vi "Service Stop Handler.vi"(8 "error in":errorcluster, 9 "stop server user event":T1, 10 "stop button ref":refnum<vi>, 11 "measurement service in":refnum<class "IMeasurement Service.lvclass">) -> (0 "error out":errorcluster, 3 "measurement service out":refnum<class "IMeasurement Service.lvclass">)   [LabVIEW 2020, in "NI Measurement Plug-In SDK.lvlib" / "IMeasurement Service.lvclass"]
uses:
  IMeasurement Service.lvclass
  Helpers/TypeDefs/Stop Server User Event.ctl
  NI Measurement Plug-In SDK.lvlib
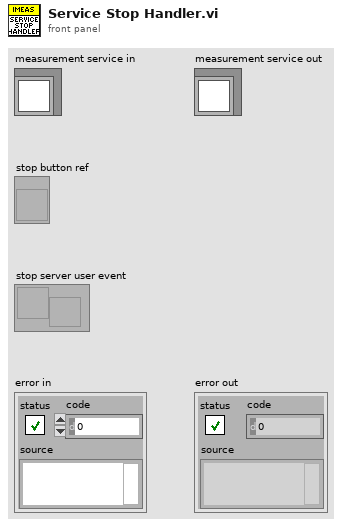
[diagram p1: front panel]
types:
  T1 = typedef "NI Measurement Plug-In SDK.lvlib/Stop Server User Event.ctl" = refnum<user-event>
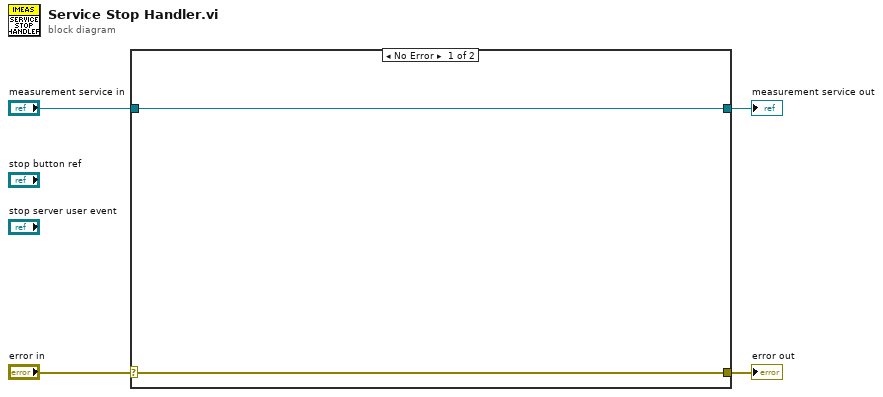
[diagram p0: block diagram]
diagram:
  n1 = case shown="No Error" "error in" {
    selector: "error in" -> [w5 w8]
    tunnel: [w5 w8] -> w3
    tunnel: [w6 w7] -> w1
    tunnel: "measurement service in" -> [w6 w7]
    frame No Error {
    }
    frame Error {
    }
  }
  "error out" <- w3
  "measurement service out" <- w1
